vi "midterm.vi"() -> ()   [LabVIEW 2023]
uses:
  <vilib>/express/express analysis/Spectral/Block/exnSpectralBlock spectral measurements RMS poly.vi
  <vilib>/express/express analysis/Spectral/Block/exnSpectralBlock spectral measurements RMS DDT.vi
  <vilib>/express/express analysis/Spectral/XNode/ExpressSpectralMeasurementsBlockNode.xnode
panel:
  in  "start_record":bool
  in  "Playback Sound":bool
  in  "Sample rate (Hz)":dbl=22050.0
  out "Most prominent frequency (Hz):":i32
  out "Frequency (logarithmic)":dynamicdata(graph)
  out "Data":dynamicdata(graph)
  in  "Duration (s)":dbl=1.0
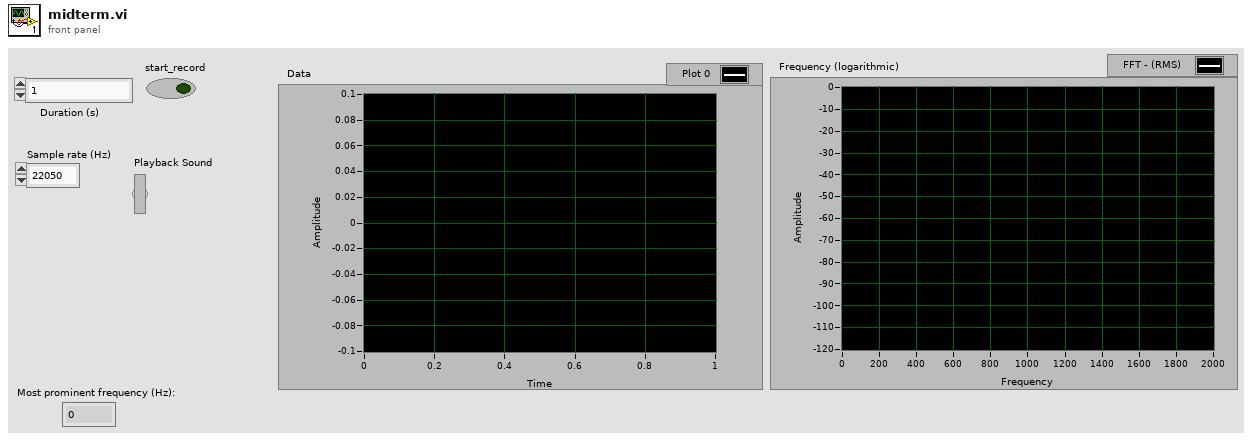
[diagram p1: front panel]
types:
  T1 = cluster{"averaging mode":u16, "weighting mode":u16, "number of averages":u32}
  T2 = cluster{"dB On (F)":bool, "unwrap phase (F)":bool, "convert to degree (F)":bool}
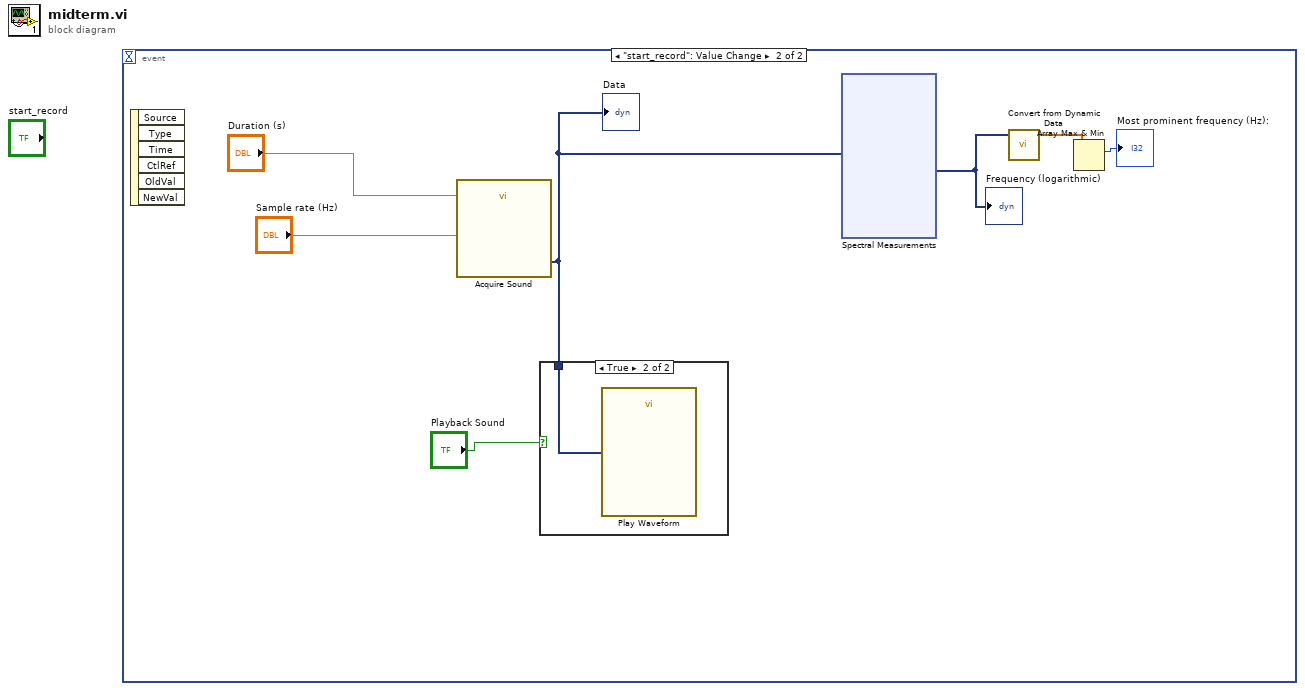
[diagram p0: block diagram]
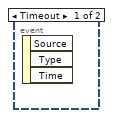
[diagram p2: hidden frame]
diagram:
  n1 = event shown="[1] \"start_record\": Value Change" {
    selector: _ -> [_ _]
    dyn-events: _ -> [_ _]
    timeout: _ -> [_ _]
    event Timeout {
      n2 = event-data() -> ()  [unwired: 1 in, 3 out]
    }
    event "start_record": Value Change {
      n3 = event-data() -> ()  [unwired: 1 in, 6 out]
      n4 = call "Acquire Sound"("Duration (s)"="Duration (s)", "Sample rate (Hz)"="Sample rate (Hz)") -> ("Data"=w1:dynamicdata)  [unwired: 16 in, 1 out]
      "Data" <- w1
      n5 = case shown="True" "Playback Sound" {
        tunnel: w1 -> [_ w8]
        frame False {
        }
        frame True {
          n6 = call "Play Waveform"("Data"=w8) -> ()  [unwired: 18 in, 1 out]
        }
      }
      n7 = xnode "Spectral Measurements"("Signals"=w1) -> ("FFT - (RMS)"=w3:dynamicdata)  [unwired: 1 in, 2 out]
      "Frequency (logarithmic)" <- w3
      n8 = call "Convert from Dynamic Data"("Dynamic Data Type"=w3) -> ("Array"=w4:dbl[])  [unwired: 3 in]
      n9 = Array Max & Min(array=w4) -> (max index (indices)=→"Most prominent frequency (Hz):":i32)  [unwired: 3 out]
    }
  }
